vi "Init.vi"(0 "object in":refnum<class "Excel.lvclass">, 2 "Data Method":refnum<class "IDataMethod.lvclass">, 5 "error in (no error)":errorcluster) -> (14 "object out":refnum<class "Excel.lvclass">, 19 "error out":errorcluster)   [LabVIEW 2024, in "Excel.lvclass"]
uses:
  Excel.lvclass
  C:/Users/burakkorkmaz/Desktop/Leveling/labview-desing-patterns/Bridge Pattern/Abstractions/DataType/DataType.lvclass
  IDataMethod_interface/IDataMethod.lvclass
  Support/Type Def/File Type.ctl
panel:
  # "Connector Pane"
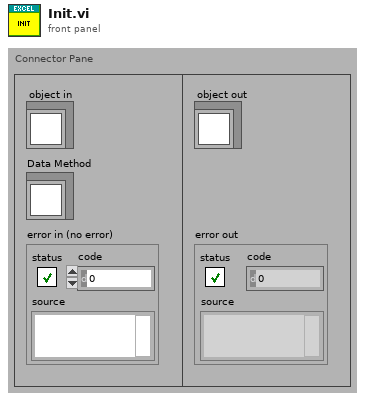
[diagram p1: front panel]
types:
  T1 = typedef "File Type.ctl" = enum32{"TDMS", "EXCEL"}
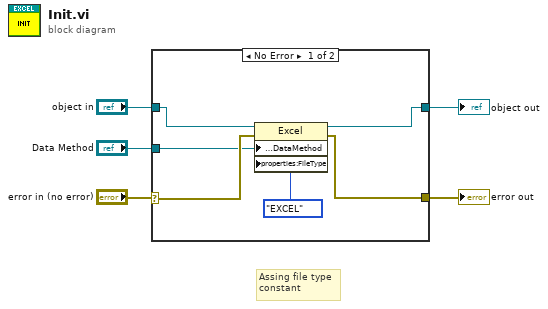
[diagram p0: block diagram]
diagram:
  # "Assing file type\nconstant"
  n1 = case shown="No Error" "error in (no error)" {
    selector: "error in (no error)" -> [w11 w12]
    tunnel: [w8 w13] -> w5
    tunnel: "object in" -> [w10 w13]
    tunnel: [w9 w12] -> w2
    tunnel: "Data Method" -> [w6 _]
    frame No Error {
      n2 = property class="Excel"(reference=w10, error in=w11, "properties:DataMethod"=w6, "properties:FileType"=File_Type."EXCEL" ("FileType")) -> (reference out=w8:refnum<class "Excel.lvclass">, error out=w9:errorcluster)
    }
    frame Error {
    }
  }
  "object out" <- w5
  "error out" <- w2
